vi "Set Current Index.vi"(8 "error in (no error)":errorcluster, 10 "Index":i32, 11 "PPT in":refnum<class "PPT.lvclass">) -> (0 "error out":errorcluster, 3 "PPT out":refnum<class "PPT.lvclass">)   [LabVIEW 2014]
uses:
  PPT.lvclass
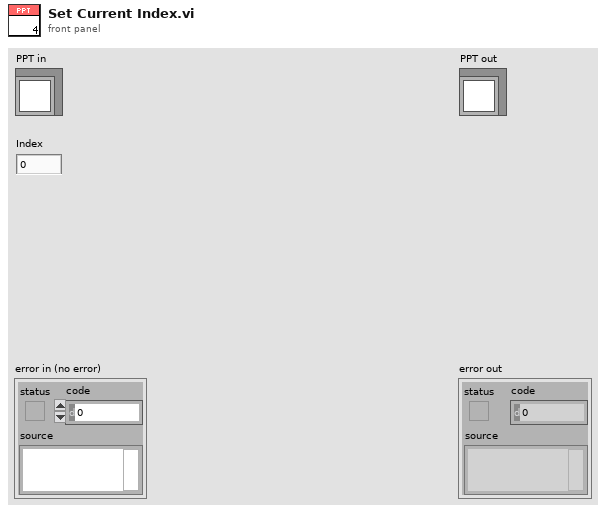
[diagram p1: front panel]
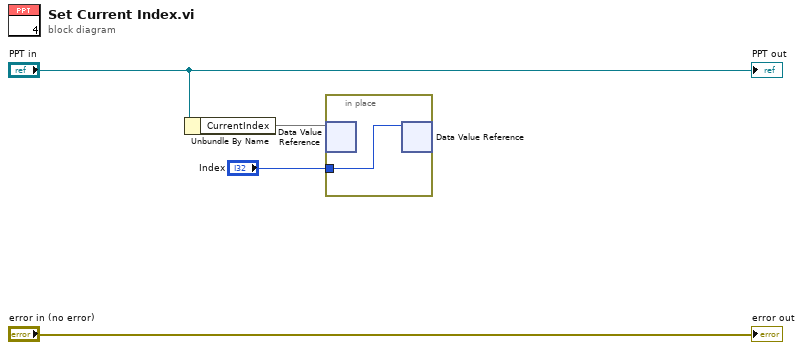
[diagram p0: block diagram]
diagram:
  n1 = Unbundle By Name("PPT in") -> ("CurrentIndex"=w2)
  n2 = in-place {
    in-place-border: "Index" -> [w5]
    n3 = in-place-dvr #1(w2) -> ()  [unwired: 2 out]
    n4 = in-place-dvr #1(w5) -> ()  [unwired: 2 out]
  }
  "error out" <- "error in (no error)"
  "PPT out" <- "PPT in"
